vi "poly_data_queue_U8.vi"(6 "initial queue element (0)":u8, 7 "initialize":bool, 8 "error in":errorcluster caption="Error in (no error)", 9 "queue length (100)":i32=100, 10 "input data point":u8) -> (0 "error out":errorcluster, 1 "eliminated element":u8, 2 "queue":u8[](array[numeric]), 4 "current length":i32)   [LabVIEW 2015, in "_average_tools_polys.lvlib"]
uses:
  _average_tools_polys.lvlib
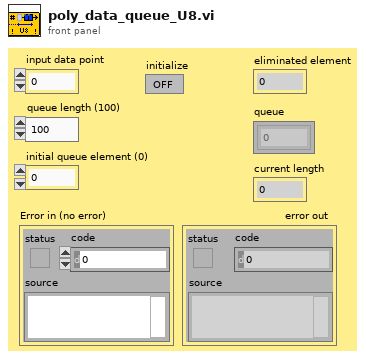
[diagram p1: front panel]
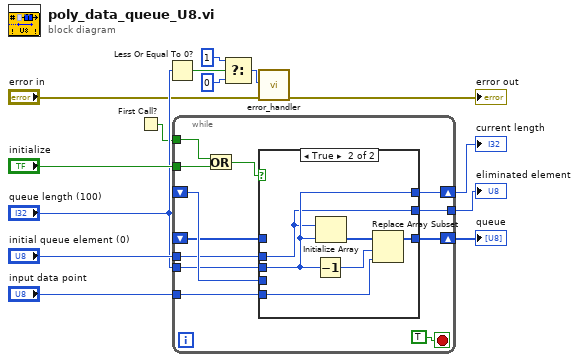
[diagram p0: block diagram]
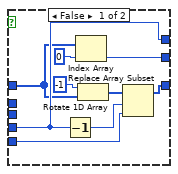
[diagram p2: hidden frame]
diagram:
  n1 = First Call?() -> (First Call?: T/F=w7:bool)
  n2 = Less Or Equal To 0?(x="queue length (100)") -> (x <= 0?=w6:bool)
  n3 = while {
    tunnel: w7 -> [w21]
    shift-left: _ -> [w24]
    shift-right: [w25] -> w13
    shift-left: _ -> [w23]
    shift-right: [w26] -> w14
    tunnel: "initialize" -> [w19]
    tunnel: "input data point" -> [w18]
    tunnel: "initial queue element (0)" -> [w17]
    tunnel: "queue length (100)" -> [w16]
    tunnel: [w15] -> w9
    stop <- TRUE stop-if-true
    n4 = Or(x=w21, y=w19) -> (x .or. y?=w20:bool)
    n5 = case shown="True" w20 {
      tunnel: [w32 w37] -> w26
      tunnel: [w33 w40] -> w25
      tunnel: w24 -> [w33 _]
      tunnel: w23 -> [w29 _]
      tunnel: w18 -> [w34 w38]
      tunnel: w17 -> [_ w36]
      tunnel: w16 -> [_ w40]
      tunnel: [w27 w36] -> w15
      frame False {
        n6 = Decrement(x=w33) -> (x-1=w31:i32)
        n7 = Index Array(array=w29, index=0 ("Index")) -> (element=w27:u8)
        n8 = Rotate 1D Array(1:w29, 2:i16 -1 ("n")) -> (0:w30:u8[])
        n9 = Replace Array Subset(array=w30, new element=w34, index=w31) -> (w32:u8[])
      }
      frame True {
        n10 = Decrement(x=w40) -> (x-1=w41:i32)
        n11 = Initialize Array(w36, w40) -> (w39:u8[])
        n12 = Replace Array Subset(array=w39, new element=w38, index=w41) -> (w37:u8[])
      }
    }
  }
  "queue" <- w14
  "current length" <- w13
  "eliminated element" <- w9
  n13 = Select(t=1, s=w6, f=0) -> (s? t:f=w3:i32)
  n14 = call "error_handler.vi"("error in (no error)"="error in", "code (0 = no error)"=w3) -> ("error out"=→"error out":errorcluster)  [unwired: 8 in, 1 out]
